vi "http_response.vi"(3 "error out 2":errorcluster, 4 "HTTP Request":T1, 5 "listener ID":refnum<k5>) -> (0 "error out":errorcluster, 1 "String":string, 2 "listener ID 2":refnum<k5>)   [LabVIEW 2011]
uses:
  http_request_response.ctl
  http_request.ctl
  http_field.ctl
  http_response.ctl
  template_field.ctl
  template_field_type.ctl
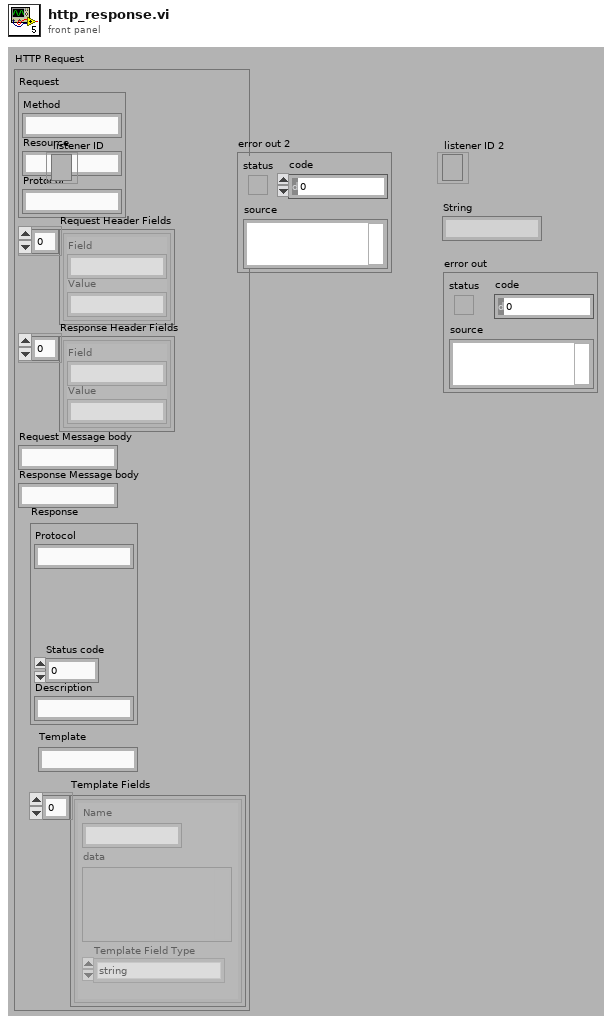
[diagram p1: front panel]
types:
  T1 = typedef "http_request_response.ctl" = cluster{"Request":T2, "Request Header Fields":T3[], "Response Header Fields":T3[], "Request Message body":string, "Response Message body":string, "Response":T4, "Template":string, "Template Fields":T5[]}
  T2 = typedef "http_request.ctl" = cluster{"Method":string, "Resource":string, "Protocol":string}
  T3 = typedef "http_field.ctl" = cluster{"Field":string, "Value":string}
  T4 = typedef "http_response.ctl" = cluster{"Protocol":string, "Status code":dbl, "Description":string}
  T5 = typedef "template_field.ctl" = cluster{"Name":string, "Template Field Type":T6, "data":variant}
  T6 = typedef "template_field_type.ctl" = enum16{"string", "string array", "number", "number array", "cluster", "cluster array"}
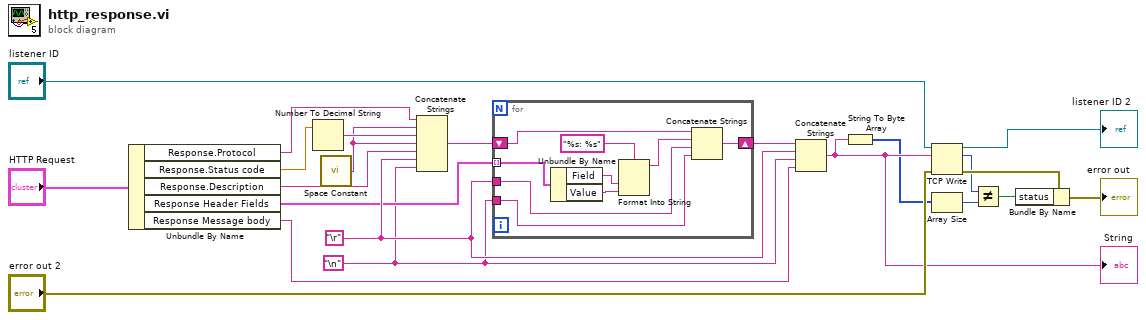
[diagram p0: block diagram]
diagram:
  w2 = "\n"
  w22 = "\r"
  n1 = Unbundle By Name("HTTP Request") -> ("Response.Protocol"=w16:string, "Response.Status code"=w15:dbl, "Response.Description"=w12:string, "Response Header Fields"=w19:T3[], "Response Message body"=w1:string)
  n2 = Number To Decimal String(number=w15) -> (decimal integer string=w14:string)  [unwired: 1 in]
  n3 = call <vilib>:"Space Constant.vi"() -> ("String"=w13:string)
  n4 = Concatenate Strings(w16, w13, w14, w13, w12, w22, w2) -> (w20:string)
  n5 = for {
    tunnel: w19 -> [w31] mode=indexing
    shift-right: [w26] -> w21
    shift-left: w20 -> [w27]
    tunnel: w22 -> [w24]
    tunnel: w2 -> [w23]
    n6 = Unbundle By Name(w31) -> ("Field"=w30:string, "Value"=w29:string)
    n7 = Format Into String(format string="%s: %s", w30, w29) -> (resulting string=w25:string)  [unwired: 2 in, 1 out]
    n8 = Concatenate Strings(w27, w25, w24, w23) -> (w26:string)
  }
  n9 = Concatenate Strings(w21, w22, w2, w1) -> (w7:string)
  "String" <- w7
  n10 = String To Byte Array(string=w7) -> (unsigned byte array=w6:u8[])
  n11 = TCP Write(connection ID="listener ID", data in=w7, error in (no error)="error out 2") -> (connection ID out=→"listener ID 2":refnum<k5>, bytes written=w8:i32, error out=w10:errorcluster)  [unwired: 1 in]
  n12 = Array Size(array=w6) -> (size(s)=w5:i32)
  n13 = Not Equal?(x=w8, y=w5) -> (x != y?=w3:bool)
  n14 = Bundle By Name(cluster=w10, "status"=w3) -> (→"error out":errorcluster)
